vi "resetNonCritical.vi"() -> (0 "error out":errorcluster)   [LabVIEW 2014]
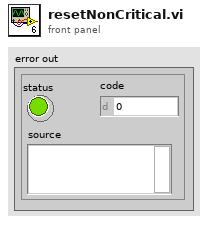
[diagram p1: front panel]
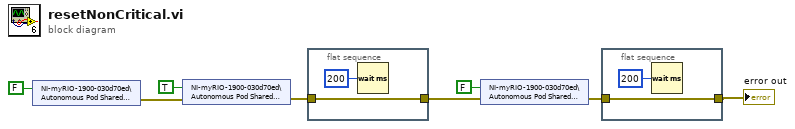
[diagram p0: block diagram]
diagram:
  n1 = shared-variable "NI-myRIO-1900-030d70ed\\Autonomous Pod Shared Variables.lvlib\\ResetSensor"(FALSE ("ResetSensor")) -> (error out=w6:errorcluster)  [unwired: 1 in]
  n2 = shared-variable "NI-myRIO-1900-030d70ed\\Autonomous Pod Shared Variables.lvlib\\SensePower"(TRUE ("SensePower"), error in=w6) -> (error out=w5:errorcluster)
  n3 = flat-sequence {
    tunnel: w5 -> [w9]
    tunnel: [w9] -> w3
    frame #0 {
      n4 = Wait (ms)(milliseconds to wait=u32 200) -> ()  [unwired: 1 out]
    }
  }
  n5 = shared-variable "NI-myRIO-1900-030d70ed\\Autonomous Pod Shared Variables.lvlib\\SensePower"(FALSE ("SensePower"), error in=w3) -> (error out=w2:errorcluster)
  n6 = flat-sequence {
    tunnel: w2 -> [w11]
    tunnel: [w11] -> w1
    frame #0 {
      n7 = Wait (ms)(milliseconds to wait=u32 200) -> ()  [unwired: 1 out]
    }
  }
  "error out" <- w1
